vi "Baseline calculation.vi"(4 "Data type":T4 items=["AXON", "HEKA"], 8 "File Paramters":T1, 9 "Sweep trace (2D) In":cluster{"Ramp Pattern":dbl[], "X":dbl[]}[][](array[cluster]), 10 "Detected Event (1D) In":cluster{dbl[][]}[](array[cluster])) -> (1 "New Baseline info":cluster{dbl[][]}[](array[cluster]), 2 "Baseline info":cluster{T3[], dbl[]}[](array[cluster]))   [LabVIEW 2017]
uses:
  Data type_new.ctl
  Baseline selection.ctl
  <vilib>/Analysis/baseanly.llb/Mean (DBL).vi
  <vilib>/Analysis/NI_AALBase.lvlib
  <vilib>/Analysis/NI_AALPro.lvlib
panel:
  out "XY 그래프":cluster{dbl[], dbl[]}[](graph)
  out "Event time":dbl
  out "Histogram Graph":T2(graph) caption="히스토그램 그래프"
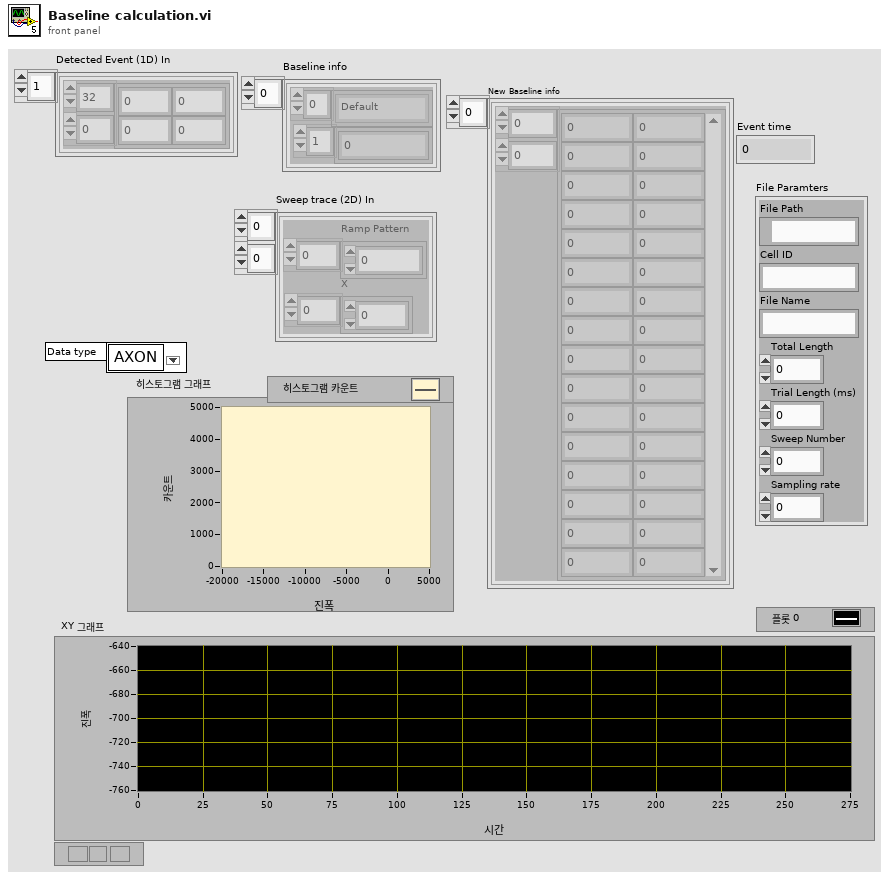
[diagram p1: front panel]
types:
  T1 = cluster{"File Path":path, "Cell ID":string, "File Name":string, "Total Length":i32, "Trial Length (ms)":dbl, "Sweep Number":dbl, "Sampling rate":dbl}
  T2 = cluster{"X Values":dbl[], "Histogram: h(x)":i32[]}
  T3 = typedef "Baseline selection.ctl" = enum16{"Default", "Manual"}
  T4 = typedef "Data type_new.ctl" = u16
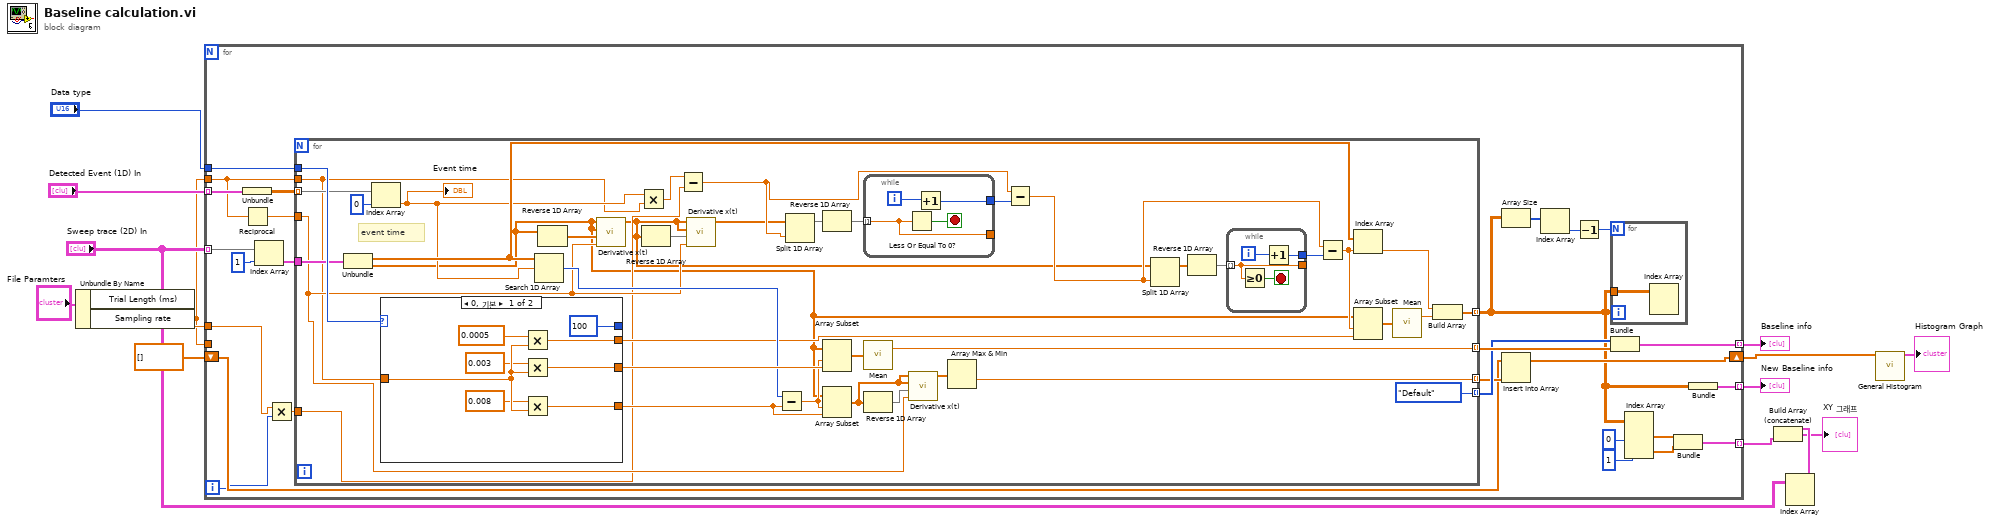
[diagram p0: block diagram]
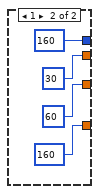
[diagram p2: hidden frame]
diagram:
  n1 = Unbundle By Name("File Paramters") -> ("Trial Length (ms)"=w4:dbl, "Sampling rate"=w1:dbl)
  n2 = for {
    tunnel: "Sweep trace (2D) In" -> [w39] mode=indexing
    tunnel: "Detected Event (1D) In" -> [w38] mode=indexing
    tunnel: [w35] -> w13 mode=indexing
    tunnel: "Data type" -> [w34]
    tunnel: [w32] -> w12 mode=indexing
    tunnel: w1 -> [w27]
    shift-right: [w30] -> w10
    shift-left: dbl[] [] -> [w29]
    tunnel: [w20] -> w8 mode=indexing
    tunnel: w4 -> [w16]
    tunnel: w1 -> [_]
    i -> [w17]
    n3 = Unbundle(w38) -> (w37:dbl[][])
    n4 = Reciprocal(x=w27) -> (1/x=w28:dbl)
    n5 = Index Array(array=w39, index=1 ("인덱스")) -> (element=w40:cluster{"Ramp Pattern":dbl[], "X":dbl[]})
    n6 = Multiply(x=w16, y=w17) -> (x*y=w15:dbl)
    n7 = for {
      tunnel: w40 -> [w55]
      tunnel: w37 -> [w57] mode=indexing
      tunnel: [w80] -> w36 mode=indexing
      tunnel: w34 -> [w82]
      tunnel: [Baseline_selection."Default" ("Baseline selection")] -> w33 mode=indexing
      tunnel: w28 -> [w54]
      tunnel: [w67] -> w23 mode=indexing
      tunnel: [w66] -> w31 mode=indexing
      tunnel: w27 -> [w49]
      tunnel: w15 -> [w52]
      # "event time"
      n8 = Unbundle(w55) -> ("Ramp Pattern"=w51:dbl[], "X"=w47:dbl[])
      n9 = Index Array(array=w57, index=0 ("인덱스")) -> (element=w50:dbl)
      "Event time" <- w50
      n10 = case shown="0, 기본" w82 {
        tunnel: [w92 160 ("y")] -> w70
        tunnel: [100 ("길이") 160 ("길이")] -> _
        tunnel: [w93 60 ("길이")] -> w79
        tunnel: [w91 30 ("길이")] -> w69
        tunnel: w49 -> [w97 _]
        frame 0, Default {
          n11 = Multiply(x=0.0005, y=w97) -> (x*y=w91:dbl)
          n12 = Multiply(x=0.003, y=w97) -> (x*y=w93:dbl)
          n13 = Multiply(x=0.008, y=w97) -> (x*y=w92:dbl)
        }
        frame 1 {
        }
      }
      n14 = Search 1D Array(1D array=w51, element=w50) -> (index of element=w77:i32)  [unwired: 1 in]
      n15 = Reverse 1D Array(array=w47) -> (reversed array=w63:dbl[])
      n16 = call <vilib>:"Derivative x(t).vi"("dt"=w54, "Final Condition"=w63, "Initial Condition"=w47, "X"=w47) -> ("dX/dt"=w43:dbl[])  [unwired: 6 in, 1 out]
      n17 = Multiply(x=w50, y=w49) -> (x*y=w53:dbl)
      n18 = Reverse 1D Array(array=w43) -> (reversed array=w62:dbl[])
      n19 = Subtract(x=w53, y=w52) -> (x-y=w48:dbl)
      n20 = call <vilib>:"Derivative x(t).vi"("dt"=w54, "Final Condition"=w62, "Initial Condition"=w43, "X"=w43) -> ("dX/dt"=w46:dbl[])  [unwired: 6 in, 1 out]
      n21 = Subtract(x=w77, y=w70) -> (x-y=w68:dbl)
      n22 = Split 1D Array(array=w46, index=w48) -> (first subarray=w61:dbl[])  [unwired: 1 out]
      n23 = Reverse 1D Array(array=w61) -> (reversed array=w60:dbl[])
      n24 = Array Subset(array=w47, index=w68, length=w79) -> (w78:dbl[])
      n25 = Array Subset(array=w47, index=w68, length=w70) -> (w76:dbl[])
      n26 = while {
        tunnel: w60 -> [w85] mode=indexing
        tunnel: [w85] -> _
        tunnel: [w83] -> w45
        i -> [w84]
        stop <- w86 stop-if-true
        n27 = Less Or Equal To 0?(x=w85) -> (x <= 0?=w86:bool)
        n28 = Increment(x=w84) -> (x+1=w83:i32)
      }
      n29 = call-poly <vilib>:"Mean.vi"("X"=w78) -> ("mean"=w80:dbl)  [unwired: 1 out]
      n30 = Reverse 1D Array(array=w76) -> (reversed array=w71:dbl[])
      n31 = call <vilib>:"Derivative x(t).vi"("dt"=w54, "Final Condition"=w71, "Initial Condition"=w76, "X"=w76) -> ("dX/dt"=w65:dbl[])  [unwired: 6 in, 1 out]
      n32 = Array Max & Min(array=w65) -> (min value=w66:dbl)  [unwired: 3 out]
      n33 = Subtract(x=w48, y=w45) -> (x-y=w44:dbl)
      n34 = Split 1D Array(array=w43, index=w44) -> (first subarray=w64:dbl[])  [unwired: 1 out]
      n35 = Reverse 1D Array(array=w64) -> (reversed array=w72:dbl[])
      n36 = while {
        tunnel: w72 -> [w89] mode=indexing
        tunnel: [w89] -> _
        tunnel: [w87] -> w59
        i -> [w88]
        stop <- w90 stop-if-true
        n37 = Greater Or Equal To 0?(x=w89) -> (x >= 0?=w90:bool)
        n38 = Increment(x=w88) -> (x+1=w87:i32)
      }
      n39 = Subtract(x=w44, y=w59) -> (x-y=w58:dbl)
      n40 = Index Array(array=w51, index=w58) -> (element=w73:dbl)
      n41 = Array Subset(array=w47, index=w58, length=w69) -> (w74:dbl[])
      n42 = call-poly <vilib>:"Mean.vi"("X"=w74) -> ("mean"=w75:dbl)  [unwired: 1 out]
      n43 = Build Array(w73, w75) -> (w67:dbl[])
    }
    n44 = Array Size(array=w23) -> (size(s)=w26:i32[])
    n45 = Insert Into Array(array=w29, new element=w31) -> (w30:dbl[])  [unwired: 1 in]
    n46 = Index Array(array=w26) -> (element=w25:i32)  [unwired: 1 in]
    n47 = Decrement(x=w25) -> (x-1=w24:i32)
    n48 = for {
      N: w24 -> [_]
      tunnel: w23 -> [w42]
      n49 = Index Array(array=w42) -> ()  [unwired: 2 in, 1 out]
    }
    n50 = Bundle(w33, w36) -> (w35:cluster{T3[], dbl[]})  [unwired: 1 in]
    n51 = Index Array(array=w23, index (col) #1=0 ("비활성화된 인덱스 (열)"), index (col) #2=1 ("인덱스 (열)")) -> (element #1=w22:dbl[], element #2=w21:dbl[])  [unwired: 2 in]
    n52 = Bundle(w22, w21) -> (w20:cluster{dbl[], dbl[]})  [unwired: 1 in]
    n53 = Bundle(w23) -> (w32:cluster{dbl[][]})  [unwired: 1 in]
  }
  "Baseline info" <- w13
  "New Baseline info" <- w12
  n54 = Index Array(array="Sweep trace (2D) In") -> (element=w7:cluster{"Ramp Pattern":dbl[], "X":dbl[]}[])  [unwired: 2 in]
  n55 = Build Array (concatenate)(w7, w8) -> (→"XY 그래프":cluster{"Ramp Pattern":dbl[], "X":dbl[]}[])
  n56 = call <vilib>:"General Histogram.vi"("X"=w10) -> ("Histogram Graph"=→"Histogram Graph":T2)  [unwired: 10 in, 4 out]
